vi "solv1.vi"(1 "Real Matrix":T1, 2 "Real Matrix (Column Vector)":T1) -> (0 "Solution Matrix":T1)   [LabVIEW 2010]
uses:
  <vilib>/Analysis/Matrix/Datatypes/RealMatrix.ctl
  <vilib>/Analysis/7linalg.llb/Real Transpose Matrix.vi
  <vilib>/Analysis/baseanly.llb/Real A x B.vi
  <vilib>/Analysis/7linalg.llb/Solve Linear Equations (multiple right hand).vi
  <vilib>/Analysis/NI_AALBase.lvlib
  <vilib>/Analysis/NI_AALPro.lvlib
  <vilib>/Analysis/Matrix/NI_Matrix.lvlib
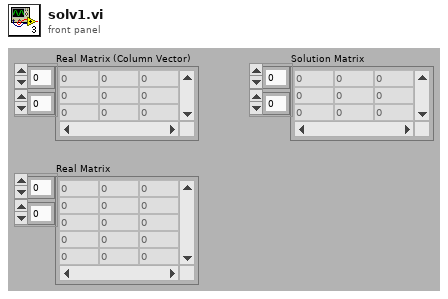
[diagram p1: front panel]
types:
  T1 = typedef "NI_Matrix.lvlib/RealMatrix.ctl" = dbl[][]
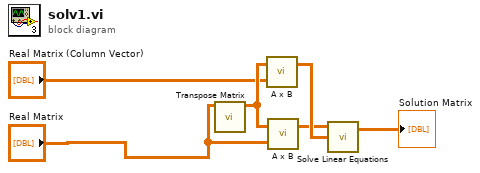
[diagram p0: block diagram]
diagram:
  n1 = call-poly <vilib>:"Transpose Matrix.vi"("Input Matrix"="Real Matrix") -> ("Matrix Transpose"=w2:T1)  [unwired: 9 in, 1 out]
  n2 = call-poly <vilib>:"A x B.vi"("B"="Real Matrix (Column Vector)", "A"=w2) -> ("A x B"=w4:T1)  [unwired: 1 out]
  n3 = call-poly <vilib>:"A x B.vi"("B"="Real Matrix", "A"=w2) -> ("A x B"=w3:T1)  [unwired: 1 out]
  n4 = call-poly <vilib>:"Solve Linear Equations.vi"("Known Matrix"=w4, "Input Matrix"=w3) -> ("Solution Matrix"=→"Solution Matrix":T1)  [unwired: 1 in, 1 out]
